vi "test.vi"() -> ()   [LabVIEW 2023]
panel:
  out "index of element":i32
  out "x+y":i32
  in  "Array":dbl[][](array[numeric])
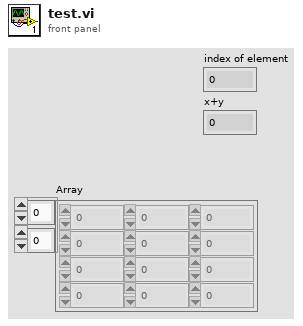
[diagram p1: front panel]
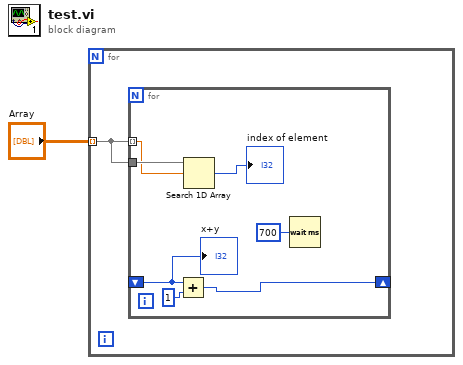
[diagram p0: block diagram]
diagram:
  n1 = for {
    tunnel: "Array" -> [w2] mode=indexing
    n2 = for {
      tunnel: w2 -> [w4] mode=indexing
      shift-right: [w7] -> _
      shift-left: _ -> [w6]
      tunnel: w2 -> [w5]
      n3 = Add(x=w6, y=1) -> (x+y=w7:i32)
      n4 = Search 1D Array(1D array=w5, element=w4) -> (index of element=→"index of element":i32)  [unwired: 1 in]
      n5 = Wait (ms)(milliseconds to wait=u32 700) -> ()  [unwired: 1 out]
      "x+y" <- w6
    }
  }
